vi "GUI_HexapodPI.vi"() -> ()   [LabVIEW 2013]
panel:
  out "indecator ref array":refnum<vi>[](array[refnum])
  in  "time to wait (TCP) 2":i32=10
  in  "plot":bool=TRUE
  out "ratio(h)":bool
  out "fixsize":bool
  in  "shotnumber":i32
  out "error (h)":bool
  out "Device Name (h)":string="StagingDG645 1"
  in  "Main Tap":T1(tab)
  in  "Stop":bool
  out "status":T2(ring) caption="HEXAPOD STATUS"
  in  "StepSize (mm)":dbl step=0.01 format="%.3f"
  in  "Wa+":bool
  in  "Wa-":bool
  in  "Ua-":bool
  in  "Va-":bool
  in  "Ua+":bool
  in  "Va+":bool
  in  "Zpos+":bool
  in  "Zpos-":bool
  in  "Xpos-":bool
  in  "YPos-":bool
  in  "XPos+":bool
  in  "YPos+":bool
  in  "uangle set":dbl caption="U Set Angle"
  out "vangle":dbl caption="V Angle"
  out "uangle":dbl caption="U Angle"
  in  "vangle set":dbl caption="V Set Angle"
  in  "xpos set":dbl caption="X Set Position"
  out "ypos":dbl caption="Y Position"
  out "xpos":dbl caption="X Position"
  in  "ypos set":dbl caption="Y Set Position"
  out "wangle":dbl caption="W Angle"
  in  "wangle set":dbl caption="W Set Angle"
  out "zpos":dbl caption="Z Position"
  in  "zpos set":dbl caption="Z Set Position"
  out "local Port":u16=65427
  out "port or service name":u16=65426
  out "Remote Host":string="192.168.11.97"
  in  "timeout ms (slow resp)":i32=500
  in  "reset":bool
  out "image con closed":bool
  out "image \nconnection":bool
  out "image con closed 2":bool=TRUE
  out "All Devices (h)":string[](array[string])=["StagingDG645 1", "StagingDG645 2"]
  in  "time to wait (TCP)":i32=10
  out "error out":errorcluster
  out "connections (hidden)":variant[](array[variant])=[variant(refnum<k16> refnum), variant(refnum<k16> refnum)]
  in  "time to wait (main loop)":i32=10
  out "Data String":string="Amplitude.Ch AB,3.000000000000\r\nAmplitude.Ch CD,4.000000000000\r\nAmplitude.Ch EF,4.000000000000\r\nAmplitude.Ch GH,4.000000000000\r\nAmplitude.Ch T0,4.000000000000\r\nDelay.Ch A,0.000000000000\r\nDelay.Ch B,0.030000000000\r\nDelay.Ch C,0.000000000000\r\nDelay.Ch D,0.030000000000\r\nDelay.Ch E,0.000000000000\r\nDelay.Ch F,0.030000000000\r\nDelay.Ch G,0.000000000000\r\nDelay.Ch H,0.030000000000\r\nDelay.Ch T0,0.000000000000\r\nDelay.Ch T1,0.030000\r\nInhibit,Triggers\r\nLinked.Ch A,T0\r\nLinked.Ch B,A\r\nLinked.Ch C,T0\r\nLinked.Ch D,C\r\nLinked.Ch E,T0\r\nLinked.Ch F,E\r\nLinked.Ch G,T0\r\nLinked.Ch H,G\r\nLocalSavingPath,c:\\temp\r\nSave,off\r\nTrigger.ExecuteSingleShot,\r\nTrigger.Level,1.000000\r\nTrigger.Rate,10.000000\r\nTrigger.Source,External rising edges\r\ntimeout,0.000000\r\nPolarity.Ch AB,Positive\r\nPolarity.Ch CD,Positive\r\nPolarity.Ch EF,Positive\r\nPolarity.Ch GH,Positive\r\nPolarity.Ch T0,Positive\r\n"
  in  "Local Saving Path":path
  out "error message":string
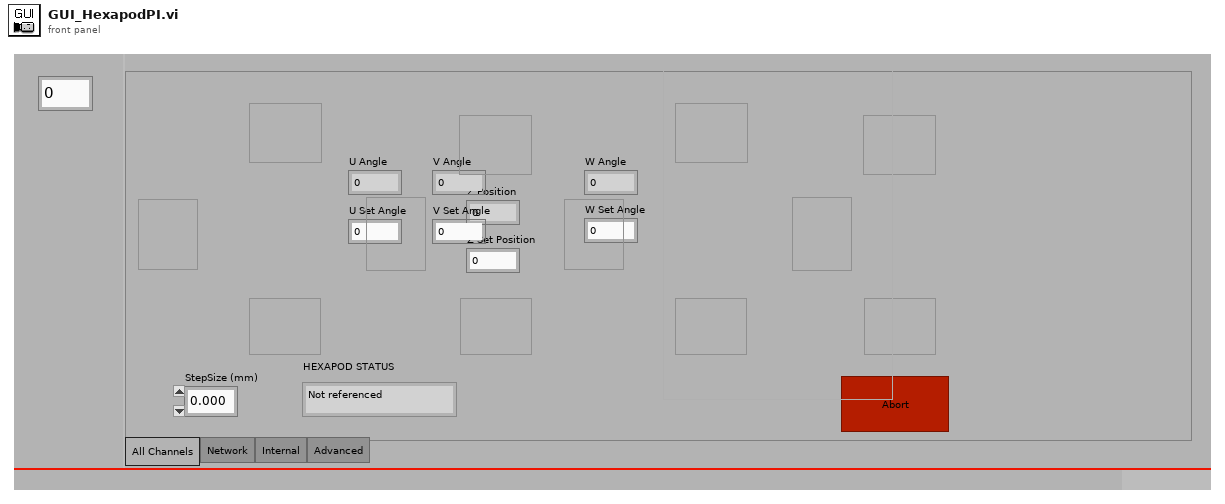
[diagram p1: front panel]
types:
  T1 = enum32{"All Channels", "Network", "Internal", "Advanced"}
  T2 = enum16{"Not referenced", "Homing", "Moving", "Ready"}
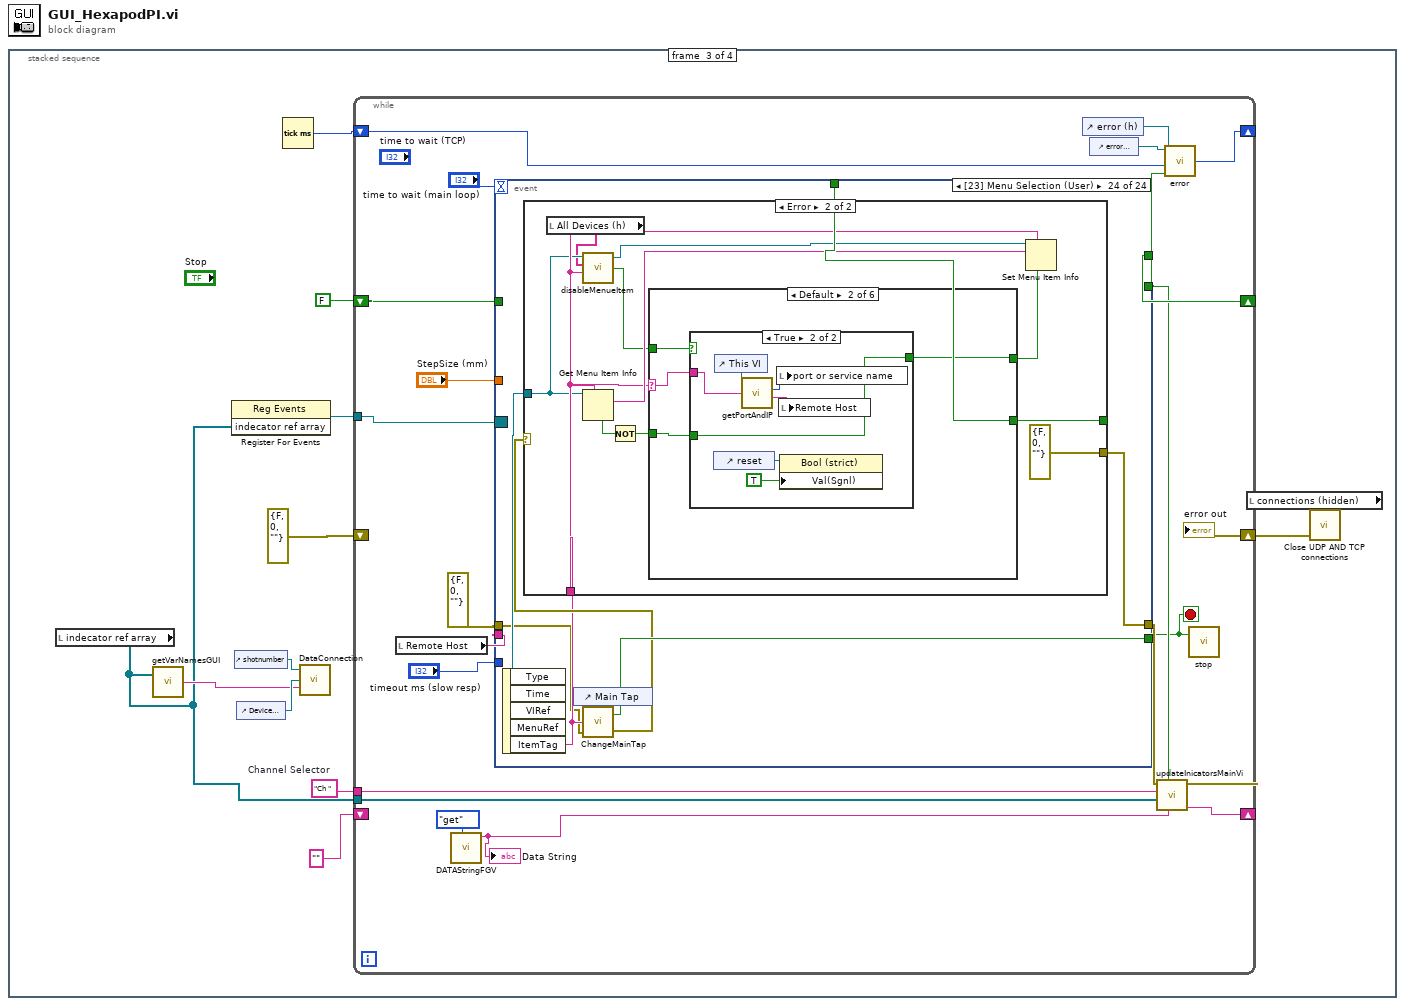
[diagram p0: block diagram]
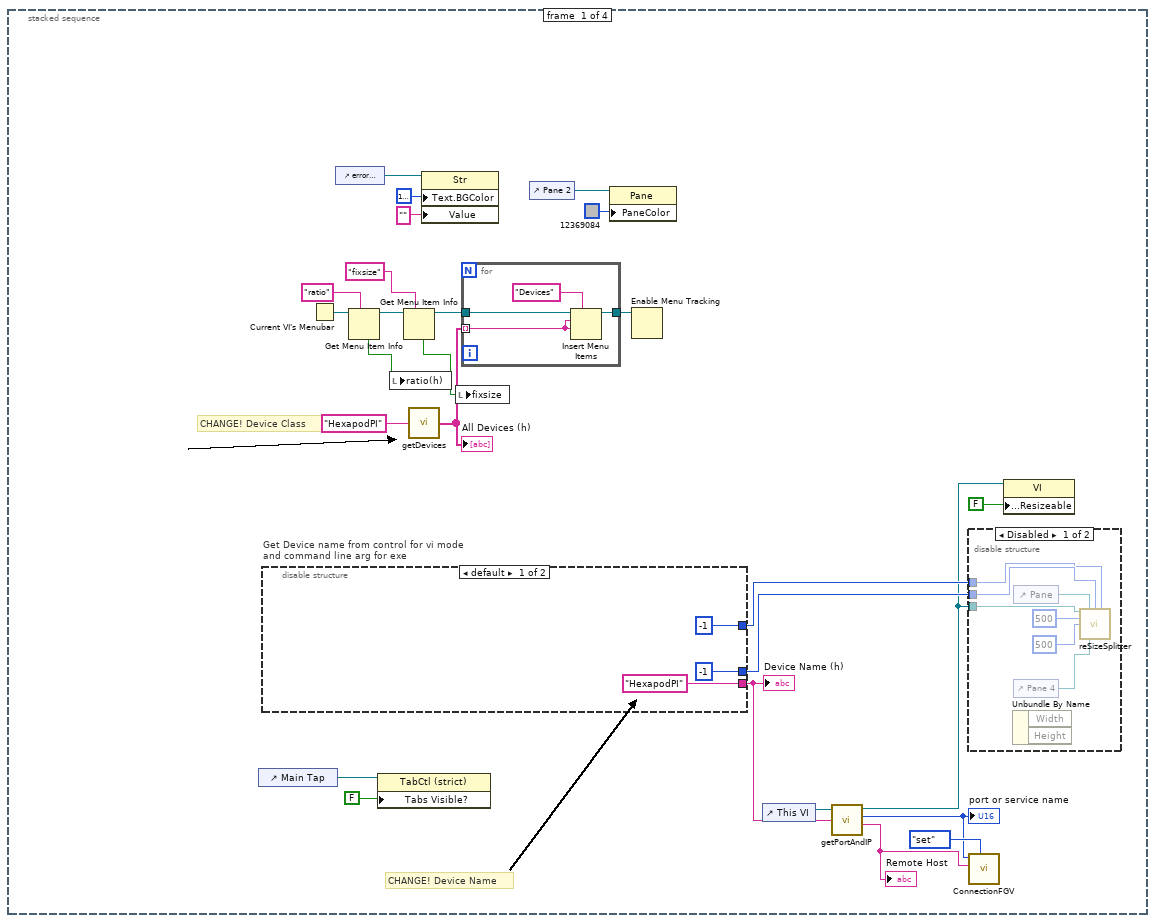
[diagram p2: hidden frame]
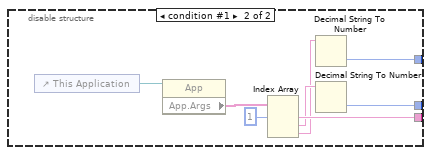
[diagram p4: hidden frame]
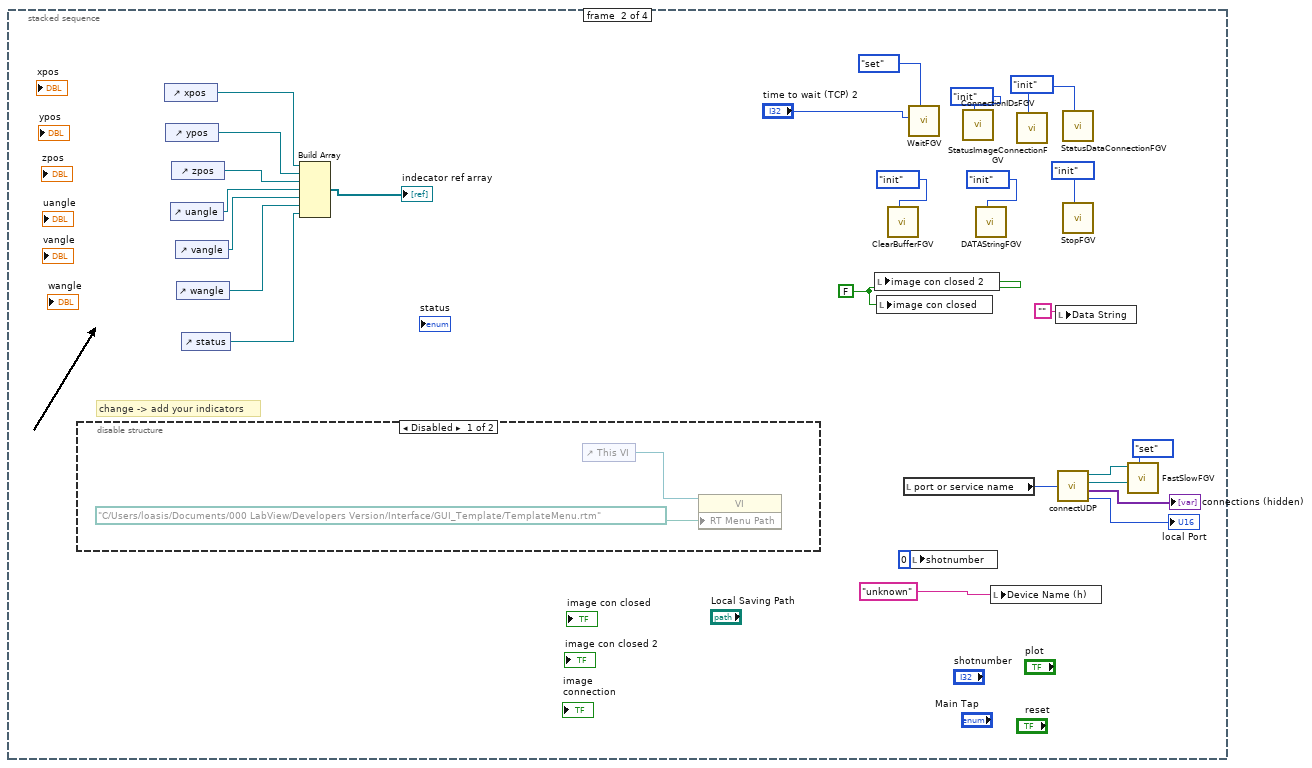
[diagram p5: hidden frame]
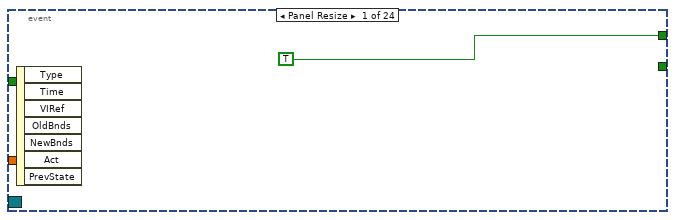
[diagram p7: hidden frame]
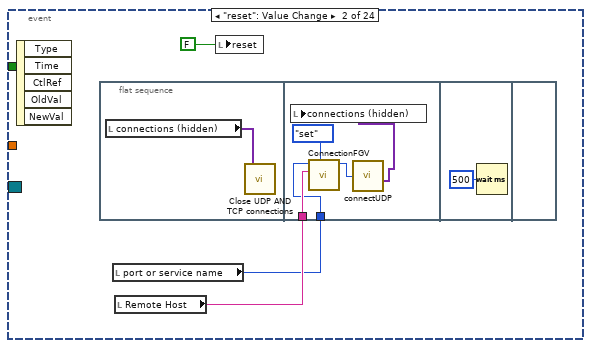
[diagram p8: hidden frame]
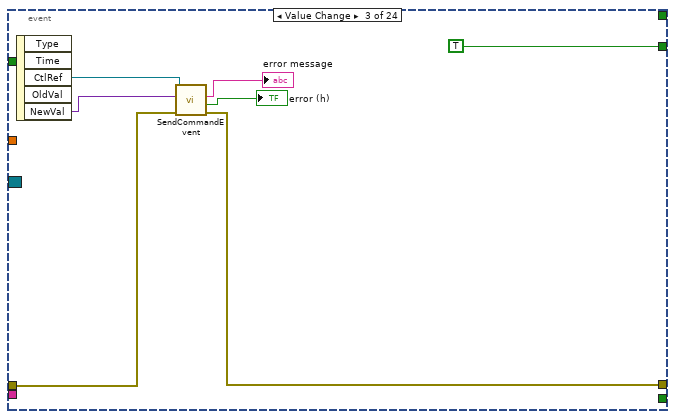
[diagram p9: hidden frame]
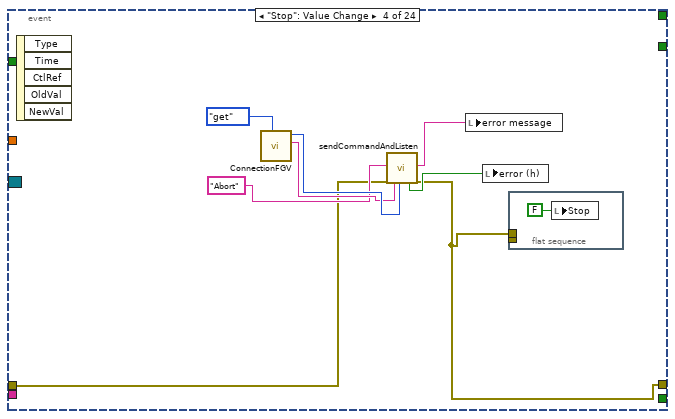
[diagram p10: hidden frame]
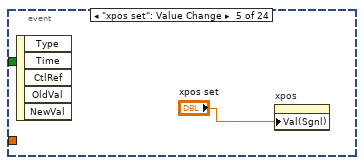
[diagram p11: hidden frame]
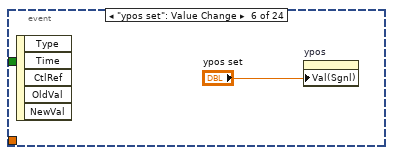
[diagram p12: hidden frame]
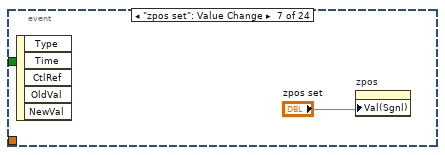
[diagram p13: hidden frame]
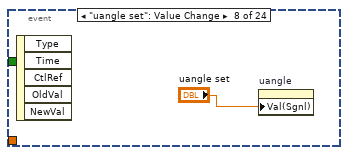
[diagram p14: hidden frame]
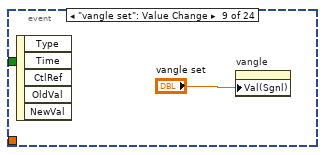
[diagram p15: hidden frame]
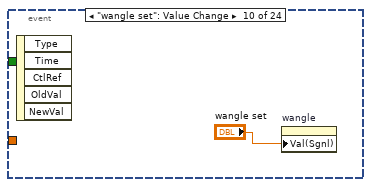
[diagram p16: hidden frame]
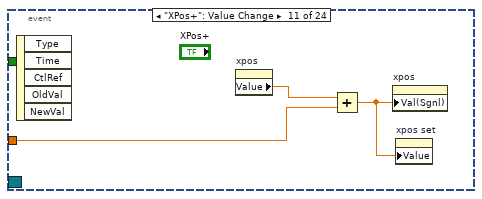
[diagram p17: hidden frame]
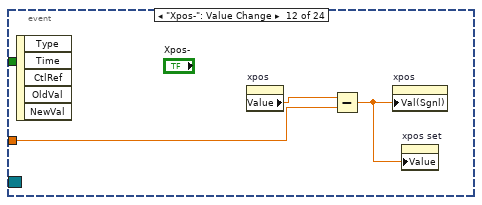
[diagram p18: hidden frame]
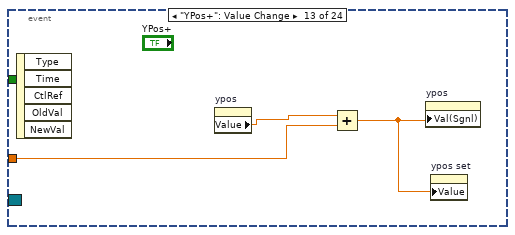
[diagram p19: hidden frame]
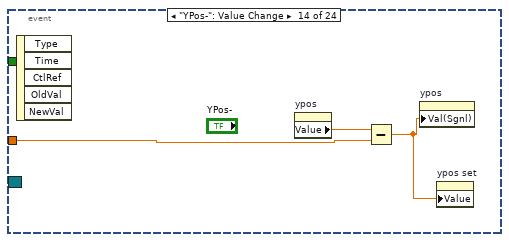
[diagram p20: hidden frame]
diagram:
  n1 = stacked-sequence {
    frame #0 {
      # "CHANGE! Device Name"
      # "CHANGE! Device Class"
      n2 = control-ref of="Main Tap"() -> (w26:refnum<vi>)
      n3 = disable-structure "Get Device name from control for vi mode\nand command line arg for exe" shown="default" {
        disable-tunnel: ["HexapodPI" ("Device Name for vi mode") w45] -> w22
        disable-tunnel: [i16 -1 ("left") w42] -> w24
        disable-tunnel: [i16 -1 ("left") w41] -> w23
        frame condition #0 (active) {
        }
        frame condition #1 {
          n4 = control-ref of="This Application"() -> (w48:refnum<vi>)
          n5 = property class="App"(reference=w48) -> ("App.Args"=w47:string[])  [unwired: 1 in, 2 out]
          n6 = Index Array(array=w47, index #1=1 ("index")) -> (element #1=w45:string, element #2=w44:string, element #3=w43:string)  [unwired: 2 in]
          n7 = Decimal String To Number(string=w43) -> (number=w41:i32)  [unwired: 2 in, 1 out]
          n8 = Decimal String To Number(string=w44) -> (number=w42:i32)  [unwired: 2 in, 1 out]
        }
      }
      "Device Name (h)" <- w22
      n9 = Current VI's Menubar() -> (w14:refnum<k9>)
      n10 = control-ref of="error message"() -> (w8:refnum<vi>)
      n11 = Get Menu Item Info(7:"ratio" ("item tag"), 11:w14) -> (3:w12:refnum<k9>, 4:w13:bool)  [unwired: 1 in, 5 out]
      n12 = property class="TabCtl (strict)"(reference=w26, "Tabs Visible?"=FALSE) -> ()  [unwired: 1 in, 2 out]
      n13 = local write "ratio(h)"(w13) -> ()
      n14 = Get Menu Item Info(7:"fixsize" ("item tag"), 11:w12) -> (3:w4:refnum<k9>, 4:w10:bool)  [unwired: 1 in, 5 out]
      n15 = call "getDevices.vi"("Device Class"="HexapodPI") -> ("All Devices"=w2:string[])
      "All Devices (h)" <- w2
      n16 = property class="Str"(reference=w8, "Text.BGColor"=u32 16777238, "Value"="") -> ()  [unwired: 1 in, 2 out]
      n17 = local write "fixsize"(w10) -> ()
      n18 = for {
        tunnel: w4 -> [w30]
        tunnel: [w29] -> w3
        tunnel: w2 -> [w27] mode=indexing
        n19 = Insert Menu Items(5:"Devices" ("menu tag"), 7:w27, 8:w27, 9:w30) -> (3:w29:refnum<k9>)  [unwired: 2 in, 2 out]
      }
      n20 = control-ref of="Pane 2"() -> (w6:refnum<vi>)
      n21 = property class="Pane"(reference=w6, "PaneColor"=u32 12369084) -> ()  [unwired: 1 in, 2 out]
      n22 = Enable Menu Tracking(4:w3) -> ()  [unwired: 2 in, 2 out]
      n23 = control-ref of="This VI"() -> (w21:refnum<vi>)
      n24 = call "getPortAndIP.vi"("Device Name"=w22, "This Vi"=w21) -> ("Remote Host"=w17:string, "port or service name"=w16:u16, "reference out"=w19:refnum<vi>)  [unwired: 2 in, 2 out]
      "port or service name" <- w16
      "Remote Host" <- w17
      n25 = disable-structure shown="Disabled" {
        disable-tunnel: w24 -> [w36 _]
        disable-tunnel: w23 -> [w35 _]
        disable-tunnel: w19 -> [w33 _]
        frame Disabled {
          n26 = Unbundle By Name() -> ()  [unwired: 1 in, 2 out]
          n27 = control-ref of="Pane"() -> (w37:refnum<vi>)
          n28 = control-ref of="Pane 4"() -> (w34:refnum<vi>)
          n29 = call "reSizeSplitter.vi"("this vi"=w33, "pane"=w37, "left"=w36, "top"=w35, "Width"=u32 500, "Height"=u32 500, "pane2"=w34) -> ()  [unwired: 8 in, 1 out]
        }
        frame Enabled {
        }
      }
      n30 = call "ConnectionFGV.vi"("command"=enum16{"get", "set", "init"}."set", "Remote Host in"=w17, "port or service name in"=w16) -> ()  [unwired: 7 in, 2 out]
      n31 = property class="VI"(reference=w19, "Front Panel.Resizeable"=FALSE ("Front Panel Window:Resizable")) -> ()  [unwired: 1 in, 2 out]
    }
    frame #1 {
      w65 = enum16{"get", "set", "init"}."init" ("Command")
      w71 = FALSE ("new Device Data")
      # "change -> add your indicators"
      n32 = disable-structure shown="Disabled" {
        frame Disabled {
          n33 = control-ref of="This VI"() -> (w75:refnum<vi>)
          n34 = property class="VI"(reference=w75, "RT Menu Path"=path "C:/Users/loasis/Documents/000 LabView/Developers Version/Interface/GUI_Template/TemplateMenu.rtm" ("Run-Time Menu Path")) -> ()  [unwired: 1 in, 2 out]
        }
        frame Enabled {
        }
      }
      n35 = control-ref of="xpos"() -> (w50:refnum<vi>)
      n36 = control-ref of="ypos"() -> (w55:refnum<vi>)
      n37 = control-ref of="uangle"() -> (w53:refnum<vi>)
      n38 = control-ref of="zpos"() -> (w54:refnum<vi>)
      n39 = control-ref of="vangle"() -> (w52:refnum<vi>)
      n40 = control-ref of="wangle"() -> (w51:refnum<vi>)
      n41 = control-ref of="status"() -> (w49:refnum<vi>)
      n42 = Build Array(w50, w55, w54, w53, w52, w51, w49) -> (→"indecator ref array":refnum<vi>[])
      n43 = local write "image con closed 2"(w71) -> ()
      n44 = local write "image con closed"(w71) -> ()
      n45 = call "ClearBufferFGV.vi"("Command"=enum16{"set", "get", "init"}."init") -> ()  [unwired: 10 in, 1 out]
      n46 = local read "port or service name"() -> (w61:u16)
      n47 = call "WaitFGV.vi"("Command"=enum16{"get", "set", "init"}."set", "milliseconds to wait"="time to wait (TCP) 2") -> ()  [unwired: 9 in, 1 out]
      n48 = local write "shotnumber"(0 ("shotnumber")) -> ()
      n49 = call "ConnectionIDsFGV.vi"("Command"=enum16{"add", "get", "init"}."init") -> ()  [unwired: 10 in, 1 out]
      n50 = call "DATAStringFGV.vi"("Command"=enum16{"get", "set", "init"}."init") -> ()  [unwired: 9 in, 2 out]
      n51 = local write "Device Name (h)"("unknown" ("Device Name")) -> ()
      n52 = call "StatusImageConnectionFGV.vi"("Command"=w65) -> ()  [unwired: 10 in, 1 out]
      n53 = local write "Data String"("") -> ()
      n54 = call "connectUDP.vi"("port or service name NOT USED"=w61) -> ("fast ID (h)"=w60:refnum<k16>, "slow ID (h)"=w59:refnum<k16>, "connections (hidden)"=→"connections (hidden)":variant[], "local Port"=→"local Port":u16)
      n55 = call "StatusDataConnectionFGV.vi"("Command"=w65) -> ()  [unwired: 10 in, 1 out]
      n56 = call "StopFGV.vi"("Command"=enum16{"set", "get", "init"}."init") -> ()  [unwired: 9 in, 2 out]
      n57 = call "FastSlowFGV.vi"("Command"=enum16{"get", "set", "init"}."set", "slow ID"=w59, "fast ID"=w60) -> ()  [unwired: 7 in, 2 out]
    }
    frame #2 {
      w78 = "Ch "  # Channel Selector
      n58 = local read "indecator ref array"() -> (w76:refnum<vi>[])
      n59 = call "getVarNamesGUI.vi"("Array"=w76) -> ("String"=w77:string)  [unwired: 1 in]
      n60 = register-events(w76) -> (reference out=w79:refnum<event-registration>)  [unwired: 2 in, 1 out]
      n61 = control-ref of="shotnumber"() -> (w81:refnum<vi>)
      n62 = control-ref of="Device Name (h)"() -> (w80:refnum<vi>)
      n63 = Tick Count (ms)() -> (millisecond timer value=w83:u32)
      n64 = call "DataConnection.vi"("Subscriber list"=w77, "Device Name (h)"=w80, "shotnumber"=w81) -> ()
      n65 = while {
        shift-right: [w104] -> w86
        shift-left: errorcluster {"status"=FALSE, "code"=0, "source"=""} ("error out") -> [_]
        tunnel: w76 -> [w98]
        shift-right: [w102] -> _
        shift-left: FALSE -> [w103]
        shift-right: [w101] -> _
        shift-left: w83 -> [w100]
        shift-right: [w91] -> _
        shift-left: "" ("Data String") -> [_]
        tunnel: w79 -> [w94]
        tunnel: w78 -> [w93]
        stop <- w95 stop-if-true
        n66 = local read "Remote Host"() -> (w106:string)
        n67 = call "DATAStringFGV.vi"("Command"=enum16{"get", "set", "init"}."get") -> ("Data String out"=w96:string)  [unwired: 9 in, 1 out]
        "Data String" <- w96
        n68 = event shown="[23] Menu Selection (User)" {
          selector: w94 -> [_ _ _ _ _ _ _ _ _ _ _ _ _ _ _ _ _ _ _ _ _ _ _ _]
          dyn-events: _ -> [_ _ _ _ _ _ _ _ _ _ _ _ _ _ _ _ _ _ _ _ _ _ _ _]
          timeout: "time to wait (main loop)" -> [_ _ _ _ _ _ _ _ _ _ _ _ _ _ _ _ _ _ _ _ _ _ _ _]
          tunnel: [_ _ w124 w127 _ _ _ _ _ _ _ _ _ _ _ _ _ _ _ _ _ _ w180 w182] -> w105
          tunnel: w106 -> [_ _ _ _ _ _ _ _ _ _ _ _ _ _ _ _ _ _ _ _ _ _ _ _]
          tunnel: "timeout ms (slow resp)" -> [_ _ _ _ _ _ _ _ _ _ _ _ _ _ _ _ _ _ _ _ _ _ _ _]
          tunnel: errorcluster {"status"=FALSE, "code"=0, "source"=""} ("error out") -> [_ _ w121 w128 _ _ _ _ _ _ _ _ _ _ _ _ _ _ _ _ _ _ w180 w183]
          tunnel: [_ _ TRUE _ _ _ _ _ _ _ _ _ _ _ _ _ _ _ _ _ _ _ _ _] -> w99
          tunnel: [_ _ _ _ _ _ _ _ _ _ _ _ _ _ _ _ _ _ _ _ _ _ _ w188] -> w95
          tunnel: [_ _ _ _ _ _ _ _ _ _ _ _ _ _ _ _ _ _ _ _ _ _ w179 w185] -> _
          tunnel: w103 -> [_ _ _ _ _ _ _ _ _ _ _ _ _ _ _ _ _ _ _ _ _ _ w179 _]
          tunnel: [TRUE _ _ _ _ _ _ _ _ _ _ _ _ _ _ _ _ _ _ _ _ _ _ _] -> w102
          tunnel: "StepSize (mm)" -> [_ _ _ _ _ _ _ _ _ _ w144 w147 w151 w153 w157 w160 w163 w166 w169 w172 w175 w178 _ _]
          event Panel Resize {
            n69 = event-data() -> ()  [unwired: 1 in, 7 out]
          }
          event "reset": Value Change {
            n70 = event-data() -> ()  [unwired: 1 in, 5 out]
            n71 = flat-sequence {
              tunnel: w111 -> [w115]
              tunnel: w110 -> [w114]
              frame #0 {
                n72 = local read "connections (hidden)"() -> (w113:variant[])
                n73 = call "Close UDP AND TCP connections.vi"("appended array"=w113) -> ()  [unwired: 7 in]
              }
              frame #1 {
                n74 = call "ConnectionFGV.vi"("command"=enum16{"get", "set", "init"}."set", "Remote Host in"=w115, "port or service name in"=w114) -> ("port or service name out"=w117:u16)  [unwired: 7 in, 1 out]
                n75 = call "connectUDP.vi"("port or service name NOT USED"=w117) -> ("connections (hidden)"=w116:variant[])  [unwired: 3 out]
                n76 = local write "connections (hidden)"(w116) -> ()
              }
              frame #2 {
                n77 = Wait (ms)(milliseconds to wait=u32 500) -> ()  [unwired: 1 out]
              }
              frame #3 {
              }
            }
            n78 = local read "port or service name"() -> (w110:u16)
            n79 = local read "Remote Host"() -> (w111:string)
            n80 = local write "reset"(FALSE ("reset")) -> ()
          }
          event Value Change {
            n81 = event-data() -> ("CtlRef"=w126:refnum<vi>, "NewVal"=w125:variant)  [unwired: 1 in, 3 out]
            n82 = call "SendCommandEvent.vi"("error out 2"=w121, "NewVal"=w125, "CtlRef"=w126) -> ("error out"=w124:errorcluster, "error (h)"=→"error (h)":bool, "error message"=→"error message":string)  [unwired: 5 in, 1 out]
          }
          event "Stop": Value Change {
            n83 = event-data() -> ()  [unwired: 1 in, 5 out]
            n84 = call "ConnectionFGV.vi"("command"=enum16{"get", "set", "init"}."get") -> ("Remote Host out"=w133:string, "port or service name out"=w134:u16)  [unwired: 9 in]
            n85 = call "sendCommandAndListen.vi"("command in"="Abort", "error in"=w128, "Remote Host"=w133, "port or service name"=w134) -> ("error"=w130:bool, "error message"=w129:string, "error out"=w127:errorcluster)  [unwired: 8 in, 5 out]
            n86 = local write "error message"(w129) -> ()
            n87 = local write "error (h)"(w130) -> ()
            n88 = flat-sequence {
              tunnel: [w135] -> _
              tunnel: w127 -> [w135]
              frame #0 {
                n89 = local write "Stop"(FALSE ("Stop")) -> ()
              }
            }
          }
          event "xpos set": Value Change {
            n90 = event-data() -> ()  [unwired: 1 in, 5 out]
            n91 = property on="xpos" class="DigNum (strict)"("Val(Sgnl)"="xpos set") -> ()  [unwired: 2 in, 2 out]
          }
          event "ypos set": Value Change {
            n92 = event-data() -> ()  [unwired: 1 in, 5 out]
            n93 = property on="ypos" class="DigNum (strict)"("Val(Sgnl)"="ypos set") -> ()  [unwired: 2 in, 2 out]
          }
          event "zpos set": Value Change {
            n94 = event-data() -> ()  [unwired: 1 in, 5 out]
            n95 = property on="zpos" class="DigNum (strict)"("Val(Sgnl)"="zpos set") -> ()  [unwired: 2 in, 2 out]
          }
          event "uangle set": Value Change {
            n96 = event-data() -> ()  [unwired: 1 in, 5 out]
            n97 = property on="uangle" class="DigNum (strict)"("Val(Sgnl)"="uangle set") -> ()  [unwired: 2 in, 2 out]
          }
          event "vangle set": Value Change {
            n98 = event-data() -> ()  [unwired: 1 in, 5 out]
            n99 = property on="vangle" class="DigNum (strict)"("Val(Sgnl)"="vangle set") -> ()  [unwired: 2 in, 2 out]
          }
          event "wangle set": Value Change {
            n100 = event-data() -> ()  [unwired: 1 in, 5 out]
            n101 = property on="wangle" class="DigNum (strict)"("Val(Sgnl)"="wangle set") -> ()  [unwired: 2 in, 2 out]
          }
          event "XPos+": Value Change {
            n102 = event-data() -> ()  [unwired: 1 in, 5 out]
            n103 = property on="xpos" class="DigNum (strict)"() -> ("Value"=w145:dbl)  [unwired: 2 in, 2 out]
            n104 = Add(x=w145, y=w144) -> (x+y=w143:dbl)
            n105 = property on="xpos" class="DigNum (strict)"("Val(Sgnl)"=w143) -> ()  [unwired: 2 in, 2 out]
            n106 = property on="xpos set" class="DigNum (strict)"("Value"=w143) -> ()  [unwired: 2 in, 2 out]
          }
          event "Xpos-": Value Change {
            n107 = event-data() -> ()  [unwired: 1 in, 5 out]
            n108 = property on="xpos" class="DigNum (strict)"() -> ("Value"=w148:dbl)  [unwired: 2 in, 2 out]
            n109 = Subtract(x=w148, y=w147) -> (x-y=w146:dbl)
            n110 = property on="xpos" class="DigNum (strict)"("Val(Sgnl)"=w146) -> ()  [unwired: 2 in, 2 out]
            n111 = property on="xpos set" class="DigNum (strict)"("Value"=w146) -> ()  [unwired: 2 in, 2 out]
          }
          event "YPos+": Value Change {
            n112 = event-data() -> ()  [unwired: 1 in, 5 out]
            n113 = property on="ypos" class="DigNum (strict)"() -> ("Value"=w150:dbl)  [unwired: 2 in, 2 out]
            n114 = Add(x=w150, y=w151) -> (x+y=w149:dbl)
            n115 = property on="ypos" class="DigNum (strict)"("Val(Sgnl)"=w149) -> ()  [unwired: 2 in, 2 out]
            n116 = property on="ypos set" class="DigNum (strict)"("Value"=w149) -> ()  [unwired: 2 in, 2 out]
          }
          event "YPos-": Value Change {
            n117 = event-data() -> ()  [unwired: 1 in, 5 out]
            n118 = property on="ypos" class="DigNum (strict)"() -> ("Value"=w154:dbl)  [unwired: 2 in, 2 out]
            n119 = Subtract(x=w154, y=w153) -> (x-y=w152:dbl)
            n120 = property on="ypos" class="DigNum (strict)"("Val(Sgnl)"=w152) -> ()  [unwired: 2 in, 2 out]
            n121 = property on="ypos set" class="DigNum (strict)"("Value"=w152) -> ()  [unwired: 2 in, 2 out]
          }
          event "Zpos+": Value Change {
            n122 = event-data() -> ()  [unwired: 1 in, 5 out]
            n123 = property on="zpos" class="DigNum (strict)"() -> ("Value"=w156:dbl)  [unwired: 2 in, 2 out]
            n124 = Add(x=w156, y=w157) -> (x+y=w155:dbl)
            n125 = property on="zpos set" class="DigNum (strict)"("Value"=w155) -> ()  [unwired: 2 in, 2 out]
            n126 = property on="zpos" class="DigNum (strict)"("Val(Sgnl)"=w155) -> ()  [unwired: 2 in, 2 out]
          }
          event "Zpos-": Value Change {
            n127 = event-data() -> ()  [unwired: 1 in, 5 out]
            n128 = property on="zpos" class="DigNum (strict)"() -> ("Value"=w159:dbl)  [unwired: 2 in, 2 out]
            n129 = Subtract(x=w159, y=w160) -> (x-y=w158:dbl)
            n130 = property on="zpos" class="DigNum (strict)"("Val(Sgnl)"=w158) -> ()  [unwired: 2 in, 2 out]
            n131 = property on="zpos set" class="DigNum (strict)"("Value"=w158) -> ()  [unwired: 2 in, 2 out]
          }
          event "Ua+": Value Change {
            n132 = event-data() -> ()  [unwired: 1 in, 5 out]
            n133 = property on="uangle" class="DigNum (strict)"() -> ("Value"=w162:dbl)  [unwired: 2 in, 2 out]
            n134 = Add(x=w162, y=w163) -> (x+y=w161:dbl)
            n135 = property on="uangle" class="DigNum (strict)"("Val(Sgnl)"=w161) -> ()  [unwired: 2 in, 2 out]
            n136 = property on="uangle set" class="DigNum (strict)"("Value"=w161) -> ()  [unwired: 2 in, 2 out]
          }
          event "Ua-": Value Change {
            n137 = event-data() -> ()  [unwired: 1 in, 5 out]
            n138 = property on="uangle" class="DigNum (strict)"() -> ("Value"=w165:dbl)  [unwired: 2 in, 2 out]
            n139 = Subtract(x=w165, y=w166) -> (x-y=w164:dbl)
            n140 = property on="uangle" class="DigNum (strict)"("Val(Sgnl)"=w164) -> ()  [unwired: 2 in, 2 out]
            n141 = property on="uangle set" class="DigNum (strict)"("Value"=w164) -> ()  [unwired: 2 in, 2 out]
          }
          event "Va+": Value Change {
            n142 = event-data() -> ()  [unwired: 1 in, 5 out]
            n143 = property on="vangle" class="DigNum (strict)"() -> ("Value"=w168:dbl)  [unwired: 2 in, 2 out]
            n144 = Add(x=w168, y=w169) -> (x+y=w167:dbl)
            n145 = property on="vangle" class="DigNum (strict)"("Val(Sgnl)"=w167) -> ()  [unwired: 2 in, 2 out]
            n146 = property on="vangle set" class="DigNum (strict)"("Value"=w167) -> ()  [unwired: 2 in, 2 out]
          }
          event "Va-": Value Change {
            n147 = event-data() -> ()  [unwired: 1 in, 5 out]
            n148 = property on="vangle" class="DigNum (strict)"() -> ("Value"=w171:dbl)  [unwired: 2 in, 2 out]
            n149 = Subtract(x=w171, y=w172) -> (x-y=w170:dbl)
            n150 = property on="vangle" class="DigNum (strict)"("Val(Sgnl)"=w170) -> ()  [unwired: 2 in, 2 out]
            n151 = property on="vangle set" class="DigNum (strict)"("Value"=w170) -> ()  [unwired: 2 in, 2 out]
          }
          event "Wa+": Value Change {
            n152 = event-data() -> ()  [unwired: 1 in, 5 out]
            n153 = property on="wangle" class="DigNum (strict)"() -> ("Value"=w174:dbl)  [unwired: 2 in, 2 out]
            n154 = Add(x=w174, y=w175) -> (x+y=w173:dbl)
            n155 = property on="wangle" class="DigNum (strict)"("Val(Sgnl)"=w173) -> ()  [unwired: 2 in, 2 out]
            n156 = property on="wangle set" class="DigNum (strict)"("Value"=w173) -> ()  [unwired: 2 in, 2 out]
          }
          event "Wa-": Value Change {
            n157 = event-data() -> ()  [unwired: 1 in, 5 out]
            n158 = property on="wangle" class="DigNum (strict)"() -> ("Value"=w177:dbl)  [unwired: 2 in, 2 out]
            n159 = Subtract(x=w177, y=w178) -> (x-y=w176:dbl)
            n160 = property on="wangle" class="DigNum (strict)"("Val(Sgnl)"=w176) -> ()  [unwired: 2 in, 2 out]
            n161 = property on="wangle set" class="DigNum (strict)"("Value"=w176) -> ()  [unwired: 2 in, 2 out]
          }
          event Timeout {
            n162 = event-data() -> ()  [unwired: 1 in, 2 out]
          }
          event Menu Selection (User) {
            n163 = event-data() -> ("MenuRef"=w184:refnum<k9>, "ItemTag"=w186:string)  [unwired: 1 in, 3 out]
            n164 = control-ref of="Main Tap"() -> (w181:refnum<vi>)
            n165 = call "ChangeMainTap.vi"("error in"=w183, "ItemTag"=w186, "reference"=w181) -> ("error out"=w187:errorcluster, "Boolean"=w188:bool)
            n166 = case shown="Error" w187 {
              selector: w187 -> [w189 _]
              tunnel: w184 -> [_ w195]
              tunnel: [_ w197] -> w185
              tunnel: w186 -> [_ w196]
              tunnel: [w189 errorcluster {"status"=FALSE, "code"=0, "source"=""} ("error IO")] -> w182
              frame No Error {
              }
              frame Error {
                n167 = local read "All Devices (h)"() -> (w190:string[])
                n168 = call "disableMenueItem.vi"("ItemTag"=w196, "All Devices (h)"=w190, "MenuRef"=w195) -> ("this is a Device(tag)"=w194:bool, "menu reference out"=w193:refnum<k9>)  [unwired: 1 in, 1 out]
                n169 = Get Menu Item Info(7:w196, 11:w195) -> (2:w199:string, 4:w200:bool)  [unwired: 1 in, 5 out]
                n170 = Not(x=w200) -> (.not. x?=w198:bool)
                n171 = case shown="Default" w196 {
                  selector: w196 -> [_ w206 _ _ _ _]
                  tunnel: w198 -> [w201 w204 w215 _ _ _]
                  tunnel: [_ _ TRUE _ _ _] -> w197
                  tunnel: w194 -> [_ w207 _ _ _ _]
                  tunnel: [w201 w205 w215 _ _ _] -> w192
                  frame "fixsize" {
                    n172 = control-ref of="This VI"() -> (w203:refnum<vi>)
                    n173 = Not(x=w201) -> (.not. x?=w202:bool)
                    n174 = property class="VI"(reference=w203, "Front Panel.Resizeable"=w202) -> ()  [unwired: 1 in, 2 out]
                    "fixsize" <- w201
                  }
                  frame Default {
                    n175 = case shown="True" w207 {
                      tunnel: w206 -> [_ w214]
                      tunnel: [_ w208] -> w205
                      tunnel: w204 -> [_ w208]
                      frame False {
                      }
                      frame True {
                        n176 = control-ref of="reset"() -> (w210:refnum<vi>)
                        n177 = control-ref of="This VI"() -> (w213:refnum<vi>)
                        n178 = call "getPortAndIP.vi"("Device Name"=w214, "This Vi"=w213) -> ("Remote Host"=w212:string, "port or service name"=w211:u16)  [unwired: 2 in, 3 out]
                        n179 = local write "port or service name"(w211) -> ()
                        n180 = local write "Remote Host"(w212) -> ()
                        n181 = property class="Bool (strict)"(reference=w210, "Val(Sgnl)"=TRUE ("Value (Signaling)")) -> ()  [unwired: 1 in, 2 out]
                      }
                    }
                  }
                  frame "ratio" {
                    "ratio(h)" <- w215
                  }
                  frame "Local Saving Path" {
                    n182 = control-ref of="Local Saving Path"() -> (w217:refnum<vi>)
                    n183 = property class="Path"(reference=w217) -> (reference out=w220:refnum<vi>, "Value"=w221:path)  [unwired: 1 in, 1 out]
                    n184 = call "changePath.vi"("Local Saving in (h)"=w221) -> ("change (h)"=w219:bool, "Local Saving out (h)"=w218:path)  [unwired: 9 in]
                    n185 = case shown="True" w219 {
                      tunnel: w220 -> [_ w223]
                      tunnel: w218 -> [_ w222]
                      frame False {
                      }
                      frame True {
                        n186 = property class="Path"(reference=w223, "Val(Sgnl)"=w222) -> ()  [unwired: 1 in, 2 out]
                      }
                    }
                  }
                  frame "reset" {
                    n187 = control-ref of="reset"() -> (w225:refnum<vi>)
                    n188 = property class="Bool (strict)"(reference=w225, "Val(Sgnl)"=TRUE ("Value (Signaling)")) -> ()  [unwired: 1 in, 2 out]
                  }
                  frame "clear" {
                    n189 = control-ref of="reset"() -> (w227:refnum<vi>)
                    n190 = property class="Bool (strict)"(reference=w227, "Val(Sgnl)"=TRUE ("Value (Signaling)")) -> ()  [unwired: 1 in, 2 out]
                  }
                }
                n191 = Set Menu Item Info(6:w192, 7:w196, 10:w199, 11:w193) -> ()  [unwired: 3 in, 2 out]
              }
            }
          }
        }
        n192 = control-ref of="error (h)"() -> (w89:refnum<vi>)
        n193 = control-ref of="error message"() -> (w90:refnum<vi>)
        n194 = call "updateInicatorsMainVi.vi"("Data String out"=w96, "Boolean"=w99, "Array"=w98, "Channel Selector"=w93, "error in"=w105) -> ("Data String out 2"=w91:string, "error out"=w104:errorcluster)  [unwired: 4 in, 1 out]
        "error out" <- w104
        n195 = call "error.vi"("Boolean"=w99, "millisecond timer value"=w100, "reference"=w89, "error message"=w90) -> ("millisecond timer value 2"=w101:u32)
        n196 = call "stop.vi"("Boolean"=w95) -> ()
      }
      n197 = local read "connections (hidden)"() -> (w85:variant[])
      n198 = call "Close UDP AND TCP connections.vi"("error in"=w86, "appended array"=w85) -> ()  [unwired: 6 in]
    }
    frame #3 {
      n199 = control-ref of="Main  Control"() -> (w229:refnum<vi>)
      n200 = property class="TabCtl (strict)"(reference=w229, "Tabs Visible?"=TRUE) -> ()  [unwired: 1 in, 2 out]
      n201 = property class="TabCtl (strict)"(reference=w229, "Tab Location"=enum32{"Top", "Bottom", "Left", "Right"}."Bottom") -> ()  [unwired: 1 in, 2 out]
      n202 = flat-sequence {
        frame #0 {
          n203 = Wait (ms)(milliseconds to wait=u32 0) -> ()  [unwired: 1 out]
        }
        frame #1 {
        }
        frame #2 {
          n204 = control-ref of="This VI"() -> (w234:refnum<vi>)
          n205 = case shown="True" FALSE {
            tunnel: w234 -> [w235 w238]
            tunnel: [w235 w236] -> w233
            frame False {
            }
            frame True {
              n206 = property class="VI" props=["Front Panel.Open"](reference=w238) -> (reference out=w237:refnum<vi>)  [unwired: 1 in, 2 out]
              n207 = invoke class="VI" method="FP.Close"(reference=w237) -> (reference out=w236:refnum<vi>)  [unwired: 2 in, 2 out]
            }
          }
          n208 = Close Reference(reference=w233) -> ()  [unwired: 1 in, 1 out]
        }
      }
    }
  }
